vi "xijk_automatic_read_table.vi"(10 "Chemin 2":path, 11 "noms des fichiers 2":string[](array[string])) -> (3 "Tableau":path[](array[path]))   [LabVIEW 2009, in "xijk_automatic_read_and_guess.lvlib"]
uses:
  xijk_automatic_read_and_guess.lvlib
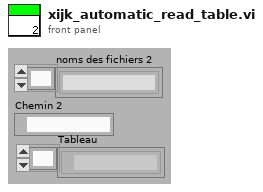
[diagram p1: front panel]
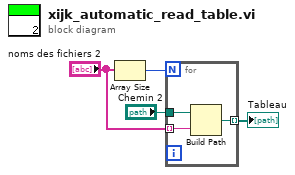
[diagram p0: block diagram]
diagram:
  n1 = Array Size(array="noms des fichiers 2") -> (size(s)=w1:i32)
  n2 = for {
    N: w1 -> [_]
    tunnel: "Chemin 2" -> [w7]
    tunnel: "noms des fichiers 2" -> [w6] mode=indexing
    tunnel: [w5] -> w3 mode=indexing
    n3 = Build Path(base path=w7, name or relative path=w6) -> (appended path=w5:path)
  }
  "Tableau" <- w3
